vi "tareatierra.vi"() -> ()   [LabVIEW 2016]
uses:
  <vilib>/picture/3D Picture Control/Object/Create Object (drawable).vi
  <vilib>/picture/3D Picture Control/Helpers/Apply Texture (no reference).vi
  <vilib>/picture/3D Picture Control/Object/Add Object (no reference).vi
  <vilib>/picture/3D Picture Control/NI_3D Picture Control.lvlib
panel:
  in  "path to JPEG file 2":path=path "C:/Program Files (x86)/National Instruments/LabVIEW 2016/examples/Graphics and Sound/3D Picture Control/pictures/earth.jpg"
  in  "z":dbl(knob) scale=0.0..360.0
  out "3D Picture":refnum<vi>(3d-picture)
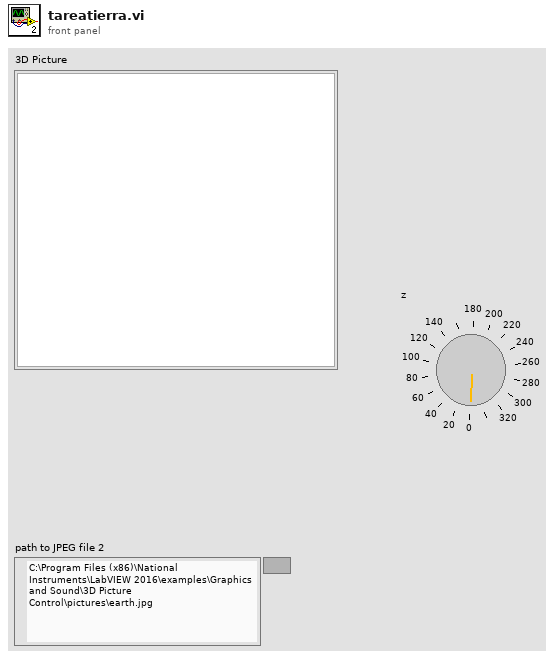
[diagram p1: front panel]
types:
  T1 = cluster{"Red":sgl, "Green":sgl, "Blue":sgl, "Alpha":sgl}
  T2 = typedef "imagedata.ctl" = cluster{"image type":i32, "image depth":i32, "image":u8[], "mask":u8[], "colors":u32[], "Rectangle":cluster{"left":i16, "top":i16, "right":i16, "bottom":i16}}
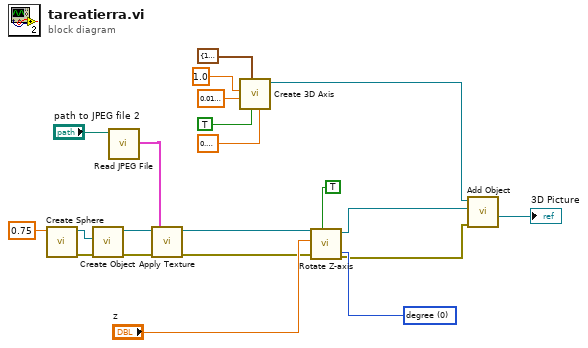
[diagram p0: block diagram]
diagram:
  w11 = u16 0 items=["degree", "radians"] ("angle unit")
  n1 = call <vilib>:"Create Sphere.vi"("Radius"=sgl 0.75) -> ("error out"=w14:errorcluster, "New Sphere Refnum"=w15:refnum<vi>)  [unwired: 9 in]
  n2 = call-poly <vilib>:"Create Object.vi"("error in (no error)"=w14, "Geometry"=w15) -> ("error out"=w5:errorcluster, "Scene:New Object"=w7:refnum<vi>)  [unwired: 8 in]
  n3 = call <vilib>:"Read JPEG File.vi"("path to JPEG file"="path to JPEG file 2") -> ("image data"=w8:T2)  [unwired: 8 in, 2 out]
  n4 = call-poly <vilib>:"Apply Texture.vi"("error in (no error)"=w5, "Image Data"=w8, "Scene Object In"=w7) -> ("error out"=w3:errorcluster, "Scene Object Out"=w4:refnum<vi>)  [unwired: 7 in]
  n5 = call <vilib>:"Create 3D Axis.vi"("Character Size"=sgl 0.2, "Axis label?"=TRUE, "Color"=T1 {"Red"=1.0, "Green"=1.0, "Blue"=1.0, "Alpha"=1.0}, "Radius"=sgl 0.02, "Length"=sgl 1.0) -> ("New Object Refnum"=w6:refnum<vi>)  [unwired: 5 in, 1 out]
  n6 = call <vilib>:"Rotate Z-axis.vi"("angle unit"=w11, "Relative?"=TRUE, "error in (no error)"=w3, "angle"="z", "Scene Object In"=w4) -> ("error out"=w1:errorcluster, "Scene Object Out"=w2:refnum<vi>)  [unwired: 5 in]
  n7 = call-poly <vilib>:"Add Object.vi"("error in (no error)"=w1, "New Object In"=w2, "Scene Object In"=w6) -> ("Scene Object Out"=→"3D Picture":refnum<vi>)  [unwired: 7 in, 1 out]
